vi "get_exe_compilation_date.vi"(8 "error_in":errorcluster) -> (0 "error_out":errorcluster, 2 "compilation_time":string="13:52", 3 "compilation_date":string="2021/12/10")   [LabVIEW 2020]
doc: "This VI allows to get exe build date and time. For it to work properly, you have to also use \"pre_build.vi\". Put \"pre_build.vi\" in \"Pre/Post Build Actions\" -> \"Execute VI before build\" in your executable build configuration."
panel:
  # "This VI allows to get exe build date and time. For it to work properly, you have to also use \"pre_build.vi\". \nPut \"pre_build.vi\" in \"Pre/Post Build Actions\" -> \"Execute VI before build\" in your executable build configuration."
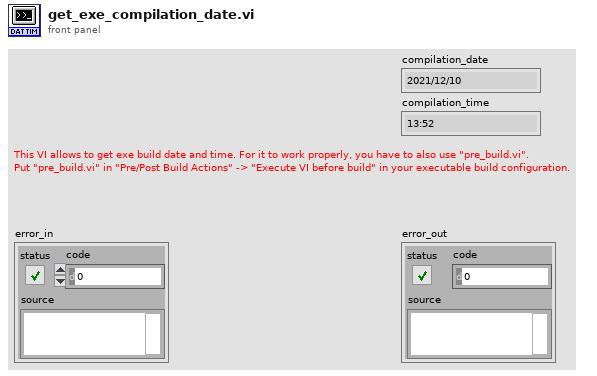
[diagram p1: front panel]
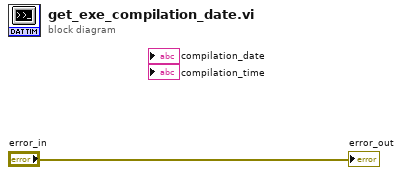
[diagram p0: block diagram]
diagram:
  "error_out" <- "error_in"
